vi "Z Stack Finish.vi"(8 "error in (no error)":errorcluster, 11 "Stage Controller in":refnum<class "Stage Controller.lvclass">) -> (0 "error out":errorcluster, 3 "Stage Controller out":refnum<class "Stage Controller.lvclass">)   [LabVIEW 2023, in "Stage Controller.lvlib" / "Stage Controller.lvclass"]
uses:
  Stage Controller.lvclass
  Stage Controller.lvclass/Stage Controller.ctl
  Resources/GLOBAL/GLOBAL Experiment Metadata.vi
  Stage Axis.ctl
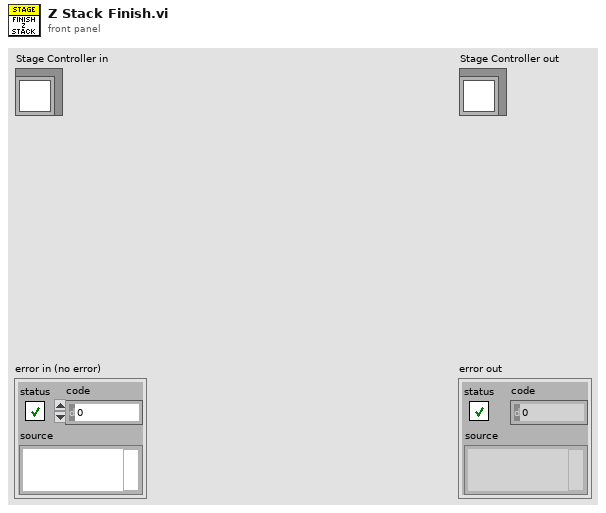
[diagram p1: front panel]
types:
  T1 = typedef "Stage Controller.lvlib/Stage Controller.lvclass/Stage Axis.ctl" = enum16{"unspecified", "X", "Y", "Z"}
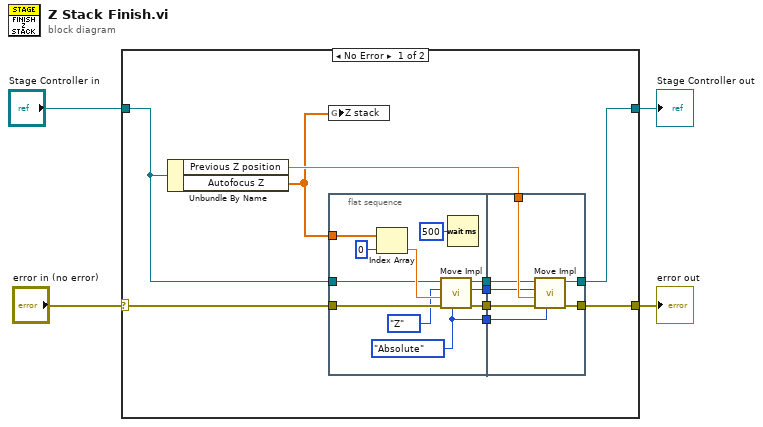
[diagram p0: block diagram]
diagram:
  n1 = case shown="No Error" "error in (no error)" {
    selector: "error in (no error)" -> [w14 w33]
    tunnel: [w12 w33] -> w3
    tunnel: [w7 w32] -> w1
    tunnel: "Stage Controller in" -> [w5 w32]
    frame No Error {
      n2 = Unbundle By Name(w5) -> ("Previous Z position"=w13:dbl, "Autofocus Z"=w6:dbl[])
      n3 = global write "GLOBAL Experiment Metadata.vi" "Z stack"(w6) -> ()
      n4 = flat-sequence "Move down first to ensure motor is engaged" {
        tunnel: w6 -> [w23]
        tunnel: w14 -> [w21]
        tunnel: [w20] -> w11
        tunnel: [w18] -> w10
        tunnel: [w17] -> w9
        tunnel: [w16] -> w8
        tunnel: w5 -> [w15]
        tunnel: w13 -> [w29]
        tunnel: [w31] -> w12
        tunnel: w11 -> [w30]
        tunnel: w10 -> [w28]
        tunnel: w9 -> [w27]
        tunnel: w8 -> [w26]
        tunnel: [w25] -> w7
        frame #0 {
          w17 = Stage_Axis."Z" ("Axis")
          w18 = enum16{"Relative", "Absolute"}."Absolute" ("Mode")
          n5 = Index Array(array=w23, index=0) -> (element=w19:dbl)
          n6 = call-dynamic "Move Impl.vi"("Mode"=w18, "error in (no error)"=w21, "Value (mm)"=w19, "Axis"=w17, "Stage Controller in"=w15) -> ("error out"=w20:errorcluster, "Stage Controller out"=w16:refnum<class "Stage Controller.lvclass">)  [unwired: 5 in]
          n7 = Wait (ms)(milliseconds to wait=u32 500) -> ()  [unwired: 1 out]
        }
        frame #1 {
          n8 = call-dynamic "Move Impl.vi"("Mode"=w28, "error in (no error)"=w30, "Value (mm)"=w29, "Axis"=w27, "Stage Controller in"=w26) -> ("error out"=w31:errorcluster, "Stage Controller out"=w25:refnum<class "Stage Controller.lvclass">)  [unwired: 5 in]
        }
      }
    }
    frame Error {
    }
  }
  "error out" <- w3
  "Stage Controller out" <- w1
